vi "Set Value.vi"(8 "error in":errorcluster, 10 "Value":variant, 11 "Cell in":refnum<class "Cell.lvclass">) -> (0 "error out":errorcluster, 3 "Cell out":refnum<class "Cell.lvclass">)   [LabVIEW 2023, in "SourceGrid.lvlib" / "Cell.lvclass"]
uses:
  Cell.lvclass
  Cell.lvclass/Cell.ctl
  D:/git/Sourcegrid-LabVIEW/dll/SourceGrid.dll
  dll/SourceGrid.dll
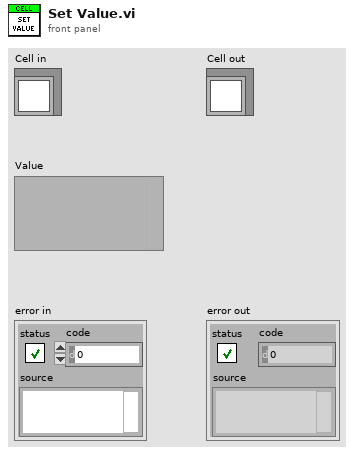
[diagram p1: front panel]
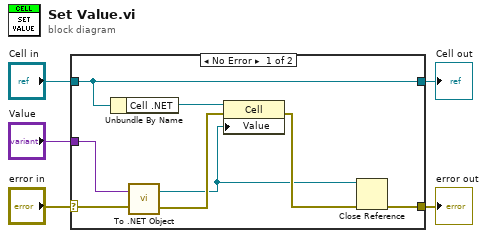
[diagram p0: block diagram]
diagram:
  n1 = case shown="No Error" "error in" {
    selector: "error in" -> [w13 w15]
    tunnel: "Cell in" -> [w6 w14]
    tunnel: "Value" -> [w11 _]
    tunnel: [w8 w15] -> w2
    tunnel: [w6 w14] -> w1
    frame No Error {
      n2 = Unbundle By Name(w6) -> ("Cell .NET"=w10:refnum<k24>)
      n3 = call <vilib>:"To .NET Object.vi"("error in (no error)"=w13, "anything"=w11) -> ("error out"=w9:errorcluster, ".NET object"=w7:refnum<k24>)
      n4 = property class="Cell"(reference=w10, error in=w9, "Value"=w7) -> (error out=w12:errorcluster)  [unwired: 1 out]
      n5 = Close Reference(reference=w7, error in (no error)=w12) -> (error out=w8:errorcluster)
    }
    frame Error {
    }
  }
  "error out" <- w2
  "Cell out" <- w1
